vi "Node v1.vi"() -> ()   [LabVIEW 2016]
uses:
  Controls/Node Data.ctl
  Controls/Node/Node - PXImc Parameters.ctl
  Controls/Node/Node - Writer Data.ctl
  Controls/Node/Node Ch Properties.ctl
  Controls/Data Type.ctl
  Controls/Node/Node - Readers Data.ctl
  Controls/Node/Node - Reader Data.ctl
  <vilib>/Utility/error.llb/DialogType.ctl
  VIs/Node/Node - Globals.vi
  PXImc Router.lvlib
panel:
  out "U8 Array Out 2":u8[](array[numeric])=[26, 21]
  out "U8 Array Out":u8[](array[numeric])=[18, 11]
  out "error out":errorcluster
  out "Numeric 4":i32=246416
  out "Numeric 3":i32=246471
  out "Numeric 2":i32=123208
  out "Numeric":i32=248409
  in  "Node 2 Data In":T1={"Node Name"="", "PXImc Parameters"={"Resource Name"="PXIMC2", "Connection Timeout (s)"=60.0, "Readers Buffer Size"=25000, "Node PXImc Reader Conn Id"=4, "Node PXImc Writer Conn Id"=3, "Writer PXImc Session"="", "Reader PXImc Session"=""}, "Local Data"={"Flattened Byte Buffer Ref"="", "Noder ID"=0, "Master Table Offest"=2, "Byte Buffer Size"=2, "Node Local Channels"=[{"Name"="", "Value"=3.0, "Data Type"=enum."U8"}, {"Name"="", "Value"=4.0, "Data Type"=enum."U8"}], "Node Local Channels Table"=[]}, "Imported Data"={"Flattened Byte Buffer Ref"="", "Byte Buffer Size"=0, "Readers Data Array"=[{"Noder ID"=0, "Master Table Offest"=0, "Byte Buffer Size"=2, "Node Imported Channels"=[{"Name"="", "Value"=0.0, "Data Type"=enum."U8"}, {"Name"="", "Value"=0.0, "Data Type"=enum."U8"}]}], "Node Imported Channels Table"=[]}}
  out "Reader Node 2":T8(graph)={"[0]"=18.0, "[1]"=26.0, "[2]"=0.0, "[3]"=0.0, "[4]"=0.0, "[5]"=0.0, "[6]"=0.0, "[7]"=0.0, "[8]"=0.0}
  out "Node 2 - Reader Ch":dbl[](array[numeric])=[18.0, 26.0]
  out "Writer Node 2":T8(graph)={"[0]"=26.0, "[1]"=21.0, "[2]"=0.0, "[3]"=0.0, "[4]"=0.0, "[5]"=0.0, "[6]"=0.0, "[7]"=0.0, "[8]"=0.0}
  in  "Node 2 - Writer Ch":dbl[](array[numeric])=[26.0, 21.0]
  out "Node 1 - Reader Ch":dbl[](array[numeric])=[21.0, 21.0]
  in  "Node 1 Data In":T1={"Node Name"="", "PXImc Parameters"={"Resource Name"="PXIMC2", "Connection Timeout (s)"=60.0, "Readers Buffer Size"=25000, "Node PXImc Reader Conn Id"=2, "Node PXImc Writer Conn Id"=1, "Writer PXImc Session"="", "Reader PXImc Session"=""}, "Local Data"={"Flattened Byte Buffer Ref"="", "Noder ID"=0, "Master Table Offest"=0, "Byte Buffer Size"=2, "Node Local Channels"=[{"Name"="", "Value"=1.0, "Data Type"=enum."U8"}, {"Name"="", "Value"=2.0, "Data Type"=enum."U8"}], "Node Local Channels Table"=[]}, "Imported Data"={"Flattened Byte Buffer Ref"="", "Byte Buffer Size"=0, "Readers Data Array"=[{"Noder ID"=0, "Master Table Offest"=2, "Byte Buffer Size"=2, "Node Imported Channels"=[{"Name"="", "Value"=0.0, "Data Type"=enum."U8"}, {"Name"="", "Value"=0.0, "Data Type"=enum."U8"}]}], "Node Imported Channels Table"=[]}}
  in  "Node 1 - Writer Ch":dbl[](array[numeric])=[18.0, 11.0]
  in  "stop":bool
  out "Writer Node 1":T8(graph)={"[0]"=18.0, "[1]"=11.0, "[2]"=0.0, "[3]"=0.0, "[4]"=0.0, "[5]"=0.0, "[6]"=0.0, "[7]"=0.0, "[8]"=0.0}
  out "Reader Node 1":T8(graph)={"[0]"=21.0, "[1]"=21.0, "[2]"=0.0, "[3]"=0.0, "[4]"=0.0, "[5]"=0.0, "[6]"=0.0, "[7]"=0.0, "[8]"=0.0}
  # "Node 1"
  # "Node 2"
  # "Node 2 => Node 1"
  # "Node 1 => Node 2"
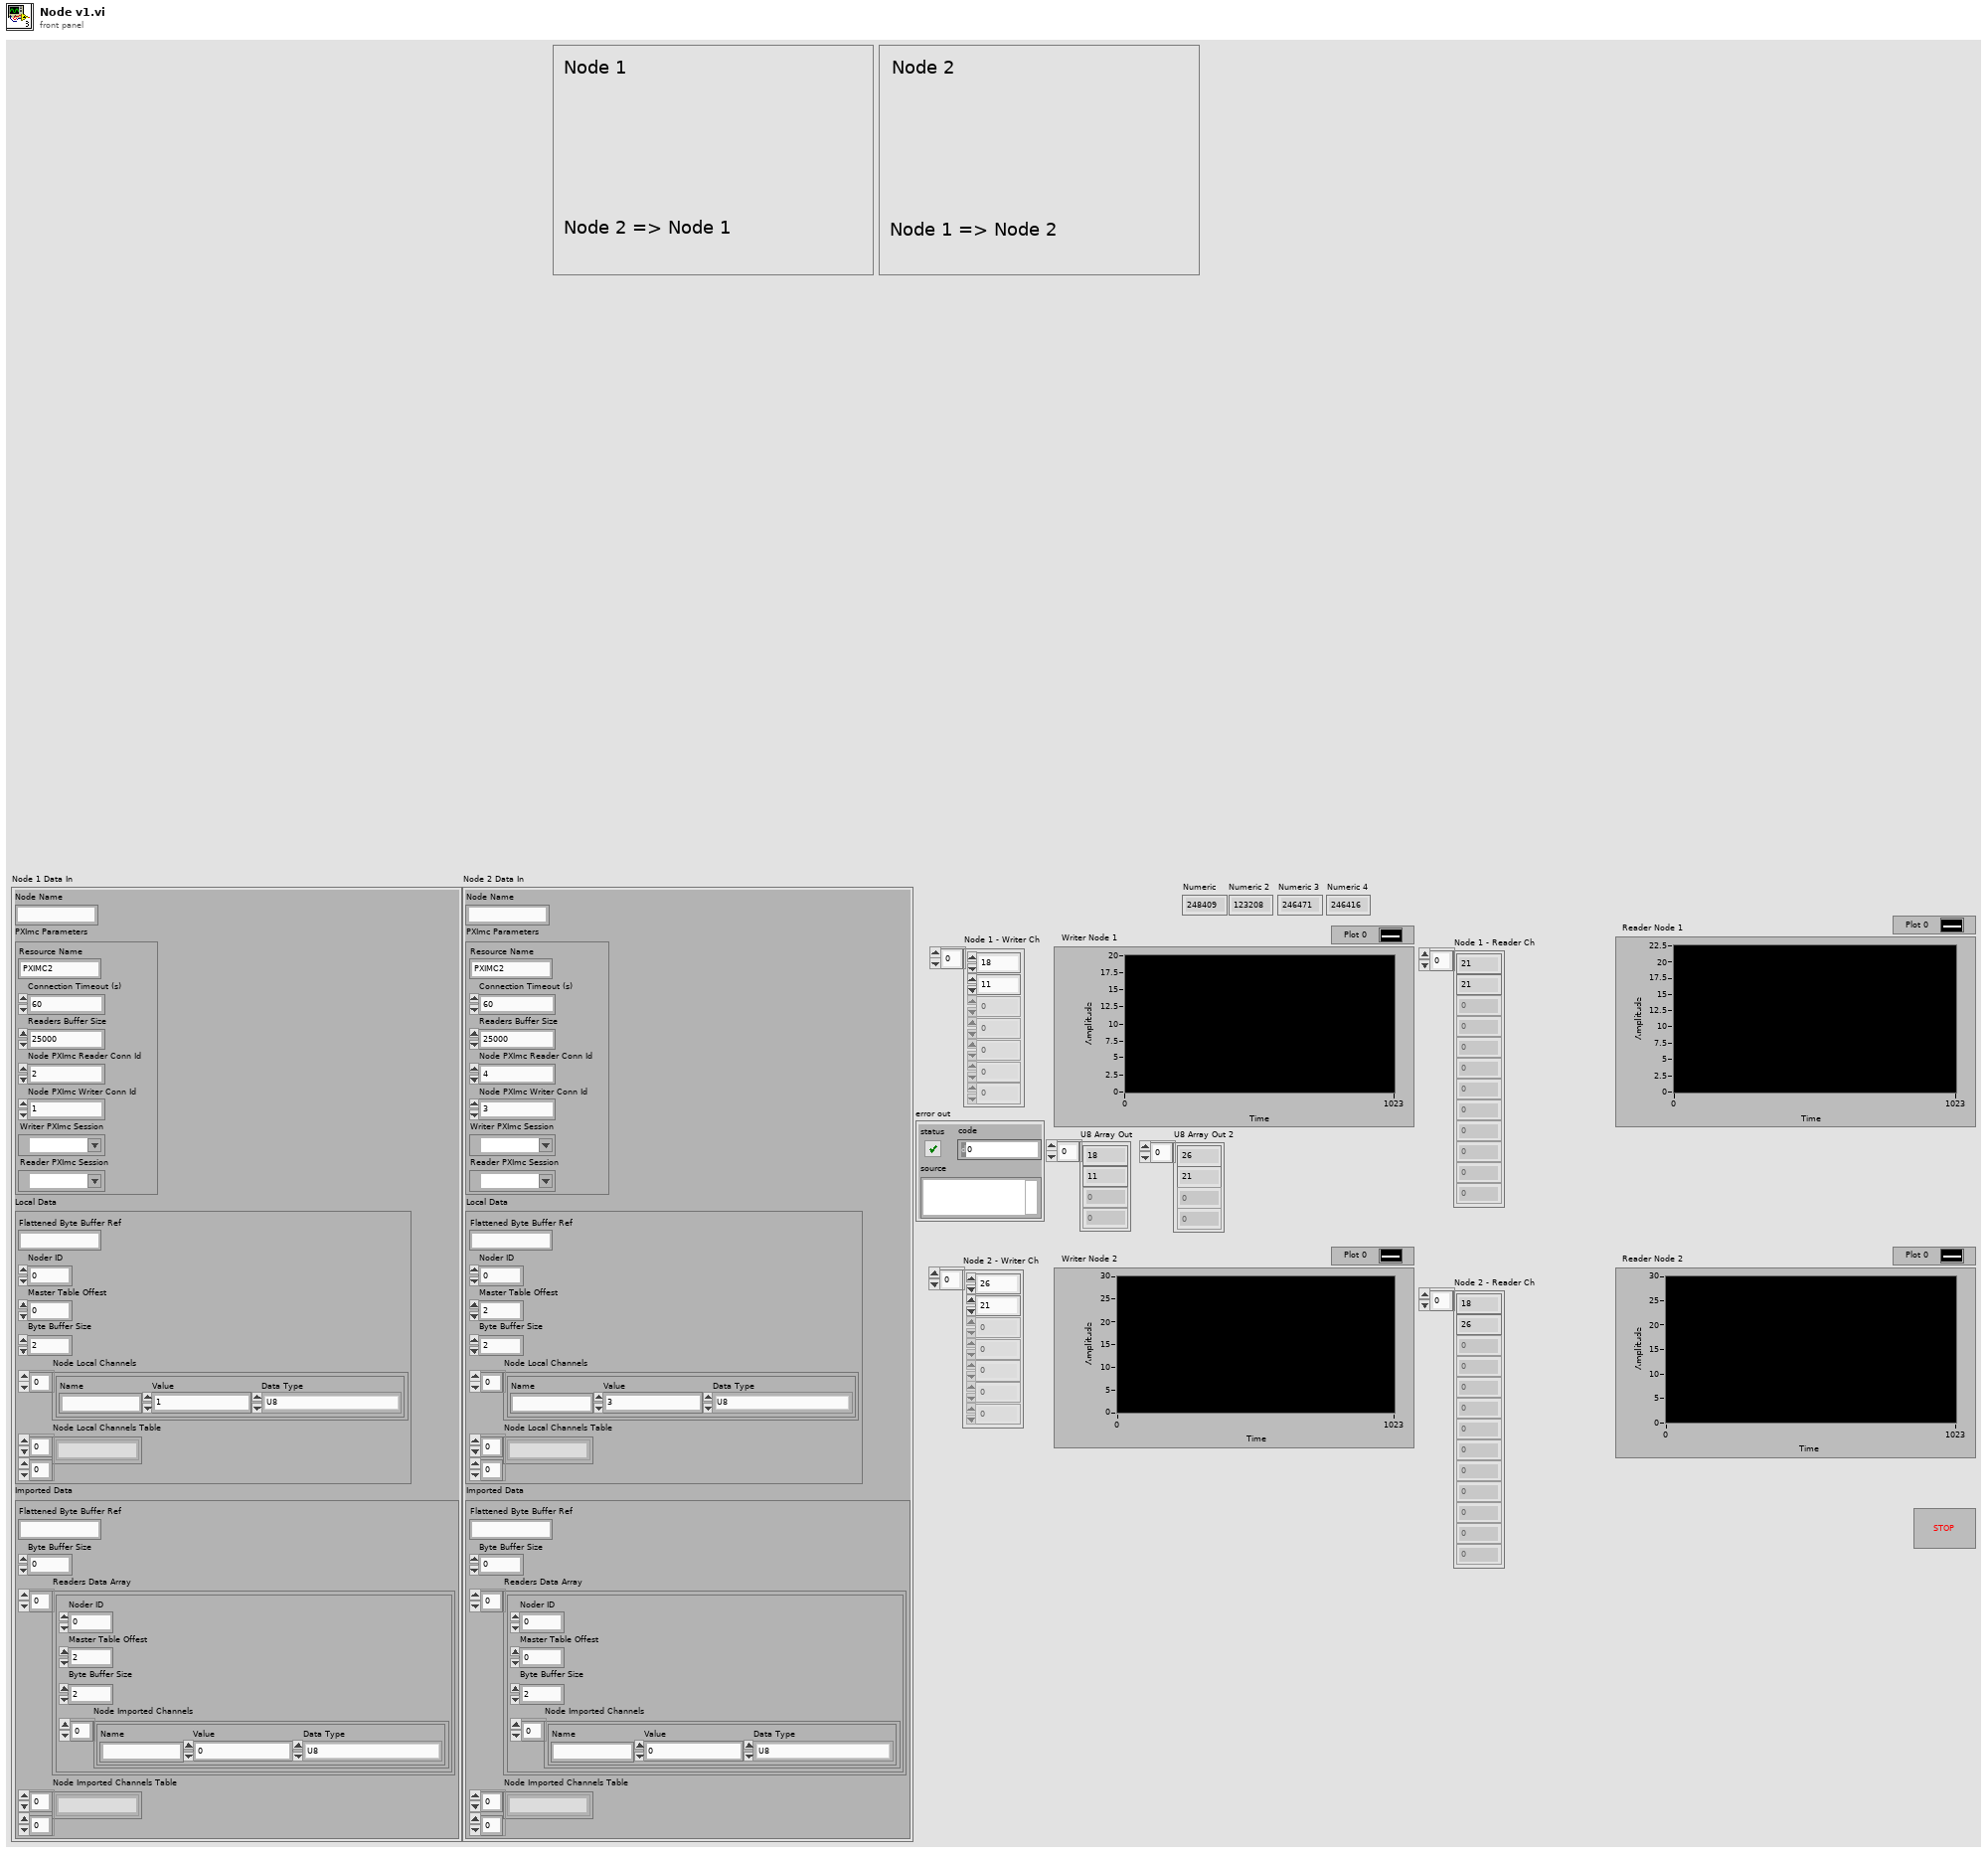
[diagram p1: front panel]
types:
  T1 = typedef "PXImc Router.lvlib/Node Data.ctl" = cluster{"Node Name":string, "PXImc Parameters":T2, "Local Data":T3, "Imported Data":T6}
  T2 = typedef "PXImc Router.lvlib/Node - PXImc Parameters.ctl" = cluster{"Resource Name":string, "Connection Timeout (s)":dbl, "Readers Buffer Size":u64, "Node PXImc Reader Conn Id":u16, "Node PXImc Writer Conn Id":u16, "Writer PXImc Session":refnum<k21>, "Reader PXImc Session":refnum<k21>}
  T3 = typedef "PXImc Router.lvlib/Node - Writer Data.ctl" = cluster{"Flattened Byte Buffer Ref":string, "Noder ID":u32, "Master Table Offest":u32, "Byte Buffer Size":u32, "Node Local Channels":T4[], "Node Local Channels Table":string[][]}
  T4 = typedef "PXImc Router.lvlib/Node Ch Properties.ctl" = cluster{"Name":string, "Value":dbl, "Data Type":T5}
  T5 = typedef "PXImc Router.lvlib/Data Type.ctl" = enum16{"Boolean", "SGL", "DBL", "I8", "I16", "I32", "I64", "U8", "U16", "U32", "U64"}
  T6 = typedef "PXImc Router.lvlib/Node - Readers Data.ctl" = cluster{"Flattened Byte Buffer Ref":string, "Byte Buffer Size":u64, "Readers Data Array":T7[], "Node Imported Channels Table":string[][]}
  T7 = typedef "PXImc Router.lvlib/Node - Reader Data.ctl" = cluster{"Noder ID":u32, "Master Table Offest":u32, "Byte Buffer Size":u64, "Node Imported Channels":T4[]}
  T8 = cluster{"[0]":dbl, "[1]":dbl, "[2]":dbl, "[3]":dbl, "[4]":dbl, "[5]":dbl, "[6]":dbl, "[7]":dbl, "[8]":dbl}
  T9 = typedef "DialogType.ctl" = u16
  T10 = cluster{"Node 1 - Writer Ch[0]":dbl, "Node 1 - Writer Ch[1]":dbl, "Node 1 - Writer Ch[2]":dbl, "Node 1 - Writer Ch[3]":dbl, "Node 1 - Writer Ch[4]":dbl, "Node 1 - Writer Ch[5]":dbl, "Node 1 - Writer Ch[6]":dbl, "Node 1 - Writer Ch[7]":dbl, "Node 1 - Writer Ch[8]":dbl}
  T11 = cluster{"Reader Ch Out[0]":dbl, "Reader Ch Out[1]":dbl, "Reader Ch Out[2]":dbl, "Reader Ch Out[3]":dbl, "Reader Ch Out[4]":dbl, "Reader Ch Out[5]":dbl, "Reader Ch Out[6]":dbl, "Reader Ch Out[7]":dbl, "Reader Ch Out[8]":dbl}
  T12 = cluster{"Node 2 - Writer Ch[0]":dbl, "Node 2 - Writer Ch[1]":dbl, "Node 2 - Writer Ch[2]":dbl, "Node 2 - Writer Ch[3]":dbl, "Node 2 - Writer Ch[4]":dbl, "Node 2 - Writer Ch[5]":dbl, "Node 2 - Writer Ch[6]":dbl, "Node 2 - Writer Ch[7]":dbl, "Node 2 - Writer Ch[8]":dbl}
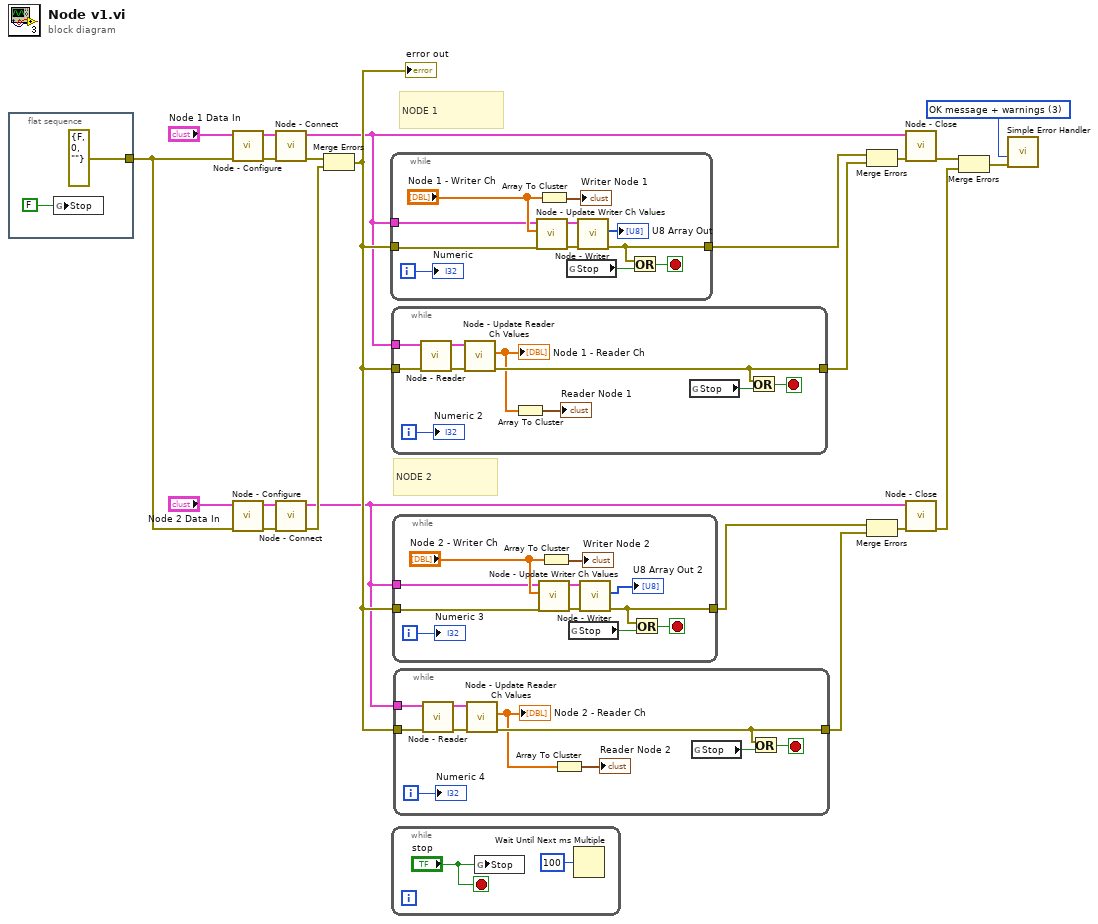
[diagram p0: block diagram]
diagram:
  w22 = T9 3 items=["no dialog", "OK message", "continue or stop message", "OK message + warnings", "continue/stop + warnings"] ("type of dialog (OK msg:1)")
  # "NODE 2"
  # "NODE 1"
  n1 = flat-sequence {
    tunnel: [errorcluster {"status"=FALSE, "code"=0, "source"=""} ("error constant")] -> w7
    frame #0 {
      n2 = global write "Node - Globals.vi" "Stop"(FALSE ("Stopped")) -> ()
    }
  }
  n3 = call "Node - Configure.vi"("error in (no error)"=w7, "Node Data In"="Node 1 Data In") -> ("error out"=w18:errorcluster, "Node Data Out"=w19:T1)  [unwired: 8 in]
  n4 = call "Node - Configure.vi"("error in (no error)"=w7, "Node Data In"="Node 2 Data In") -> ("error out"=w11:errorcluster, "Node Data Out"=w10:T1)  [unwired: 8 in]
  n5 = call "Node - Connect.vi"("error in (no error)"=w18, "Node Data In"=w19) -> ("error out"=w17:errorcluster, "Node Data Out"=w1:T1)  [unwired: 8 in]
  n6 = call "Node - Connect.vi"("error in (no error)"=w11, "Node Data In"=w10) -> ("error out"=w8:errorcluster, "Node Data Out"=w5:T1)  [unwired: 8 in]
  n7 = Merge Errors(w17, w8) -> (w9:errorcluster)
  "error out" <- w9
  n8 = while {
    tunnel: w1 -> [w30]
    tunnel: w9 -> [w29]
    tunnel: [w33] -> w21
    i -> [w26]
    stop <- w34 stop-if-true
    n9 = call "Node - Update Writer Ch Values.vi"("error in (no error)"=w29, "Writer Channels In"="Node 1 - Writer Ch", "Node Data In"=w30) -> ("error out"=w27:errorcluster, "Node Data Out"=w28:T1)  [unwired: 7 in]
    n10 = Array To Cluster(array="Node 1 - Writer Ch") -> (cluster=→"Writer Node 1":T10)
    n11 = global read "Node - Globals.vi" "Stop"() -> (w35:bool)
    n12 = call "Node - Writer.vi"("error in (no error)"=w27, "Node Data In"=w28) -> ("error out"=w33:errorcluster, "U8 Array Out"=→"U8 Array Out":u8[])  [unwired: 7 in, 1 out]
    n13 = Or(x=w33, y=w35) -> (x .or. y?=w34:bool)
    "Numeric" <- w26
  }
  n14 = while {
    tunnel: w1 -> [w41]
    tunnel: w9 -> [w45]
    tunnel: [w38] -> w20
    i -> [w36]
    stop <- w43 stop-if-true
    n15 = call "Node - Reader.vi"("error in (no error)"=w45, "Node Data In"=w41) -> ("error out"=w39:errorcluster, "Node Data Out"=w40:T1)  [unwired: 8 in]
    n16 = call "Node - Update Reader Ch Values.vi"("error in (no error)"=w39, "Node Data In"=w40) -> ("error out"=w38:errorcluster, "Reader Ch Out"=w37:dbl[])  [unwired: 7 in, 1 out]
    "Node 1 - Reader Ch" <- w37
    n17 = Array To Cluster(array=w37) -> (cluster=→"Reader Node 1":T11)
    n18 = global read "Node - Globals.vi" "Stop"() -> (w44:bool)
    n19 = Or(x=w38, y=w44) -> (x .or. y?=w43:bool)
    "Numeric 2" <- w36
  }
  n20 = while {
    stop <- "stop" stop-if-true
    n21 = global write "Node - Globals.vi" "Stop"("stop") -> ()
    n22 = Wait Until Next ms Multiple(millisecond multiple=u32 100) -> ()  [unwired: 1 out]
  }
  n23 = while {
    tunnel: w5 -> [w53]
    tunnel: w9 -> [w52]
    tunnel: [w56] -> w4
    i -> [w49]
    stop <- w57 stop-if-true
    n24 = call "Node - Update Writer Ch Values.vi"("error in (no error)"=w52, "Writer Channels In"="Node 2 - Writer Ch", "Node Data In"=w53) -> ("error out"=w50:errorcluster, "Node Data Out"=w51:T1)  [unwired: 7 in]
    n25 = Array To Cluster(array="Node 2 - Writer Ch") -> (cluster=→"Writer Node 2":T12)
    n26 = global read "Node - Globals.vi" "Stop"() -> (w58:bool)
    n27 = call "Node - Writer.vi"("error in (no error)"=w50, "Node Data In"=w51) -> ("error out"=w56:errorcluster, "U8 Array Out"=→"U8 Array Out 2":u8[])  [unwired: 7 in, 1 out]
    n28 = Or(x=w56, y=w58) -> (x .or. y?=w57:bool)
    "Numeric 3" <- w49
  }
  n29 = while {
    tunnel: w5 -> [w64]
    tunnel: w9 -> [w68]
    tunnel: [w61] -> w3
    i -> [w59]
    stop <- w66 stop-if-true
    n30 = call "Node - Reader.vi"("error in (no error)"=w68, "Node Data In"=w64) -> ("error out"=w62:errorcluster, "Node Data Out"=w63:T1)  [unwired: 8 in]
    n31 = call "Node - Update Reader Ch Values.vi"("error in (no error)"=w62, "Node Data In"=w63) -> ("error out"=w61:errorcluster, "Reader Ch Out"=w60:dbl[])  [unwired: 7 in, 1 out]
    "Node 2 - Reader Ch" <- w60
    n32 = Array To Cluster(array=w60) -> (cluster=→"Reader Node 2":T11)
    n33 = global read "Node - Globals.vi" "Stop"() -> (w67:bool)
    n34 = Or(x=w61, y=w67) -> (x .or. y?=w66:bool)
    "Numeric 4" <- w59
  }
  n35 = Merge Errors(w21, w20) -> (w16:errorcluster)
  n36 = Merge Errors(w4, w3) -> (w6:errorcluster)
  n37 = call "Node - Close.vi"("error in (no error)"=w16, "Node Data In"=w1) -> ("error out"=w15:errorcluster)  [unwired: 9 in]
  n38 = call "Node - Close.vi"("error in (no error)"=w6, "Node Data In"=w5) -> ("error out"=w2:errorcluster)  [unwired: 9 in]
  n39 = Merge Errors(w15, w2) -> (w14:errorcluster)
  n40 = call <vilib>:"Simple Error Handler.vi"("type of dialog (OK msg:1)"=w22, "error in (no error)"=w14) -> ()  [unwired: 3 in, 5 out]
